vi "Chroma Driver GPIB-VISA-RW.vi"(0 "VISA resource name":refnum<visa-resource-name>="CHROMA", 5 "Chroma Power Select":T1, 9 "Write Buffer":string="SENS:DATA?", 11 "error in (no error)":errorcluster) -> (6 "Read Array":string[](array[string]), 15 "error out":errorcluster)   [LabVIEW 2012]
doc: "This example requires NI-488.2 and NI-VISA to be installed on the system. The example shows how to communicate with a GPIB instrument using VISA reads, writes, and formatting functions on the returned data. This example will work using an NI Instrument Simulator or other instrument that has similar behavior."
uses:
  Chroma Driver Select.ctl
  <vilib>/Instr/_visa.llb/VISA Open Access Mode.ctl
panel:
  out "Array":errorcluster[](array[cluster])
  out "Success":bool
  out "Read Buffer":string
  # "Voltage \nPower\nCurrent \nState\nPhase\nError?"
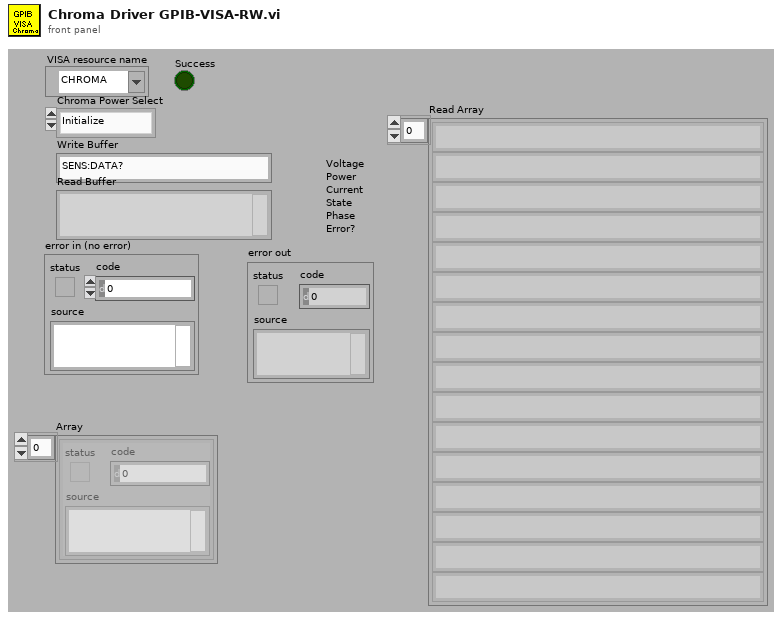
[diagram p1: front panel]
types:
  T1 = typedef "Chroma Driver Select.ctl" = enum16{"Initialize", "Output On 120", "Output On 240", "Output On 208", "Output Off", "Status", "Send Command", "Track Current"}
  T2 = typedef "VISA Open Access Mode.ctl" = u32
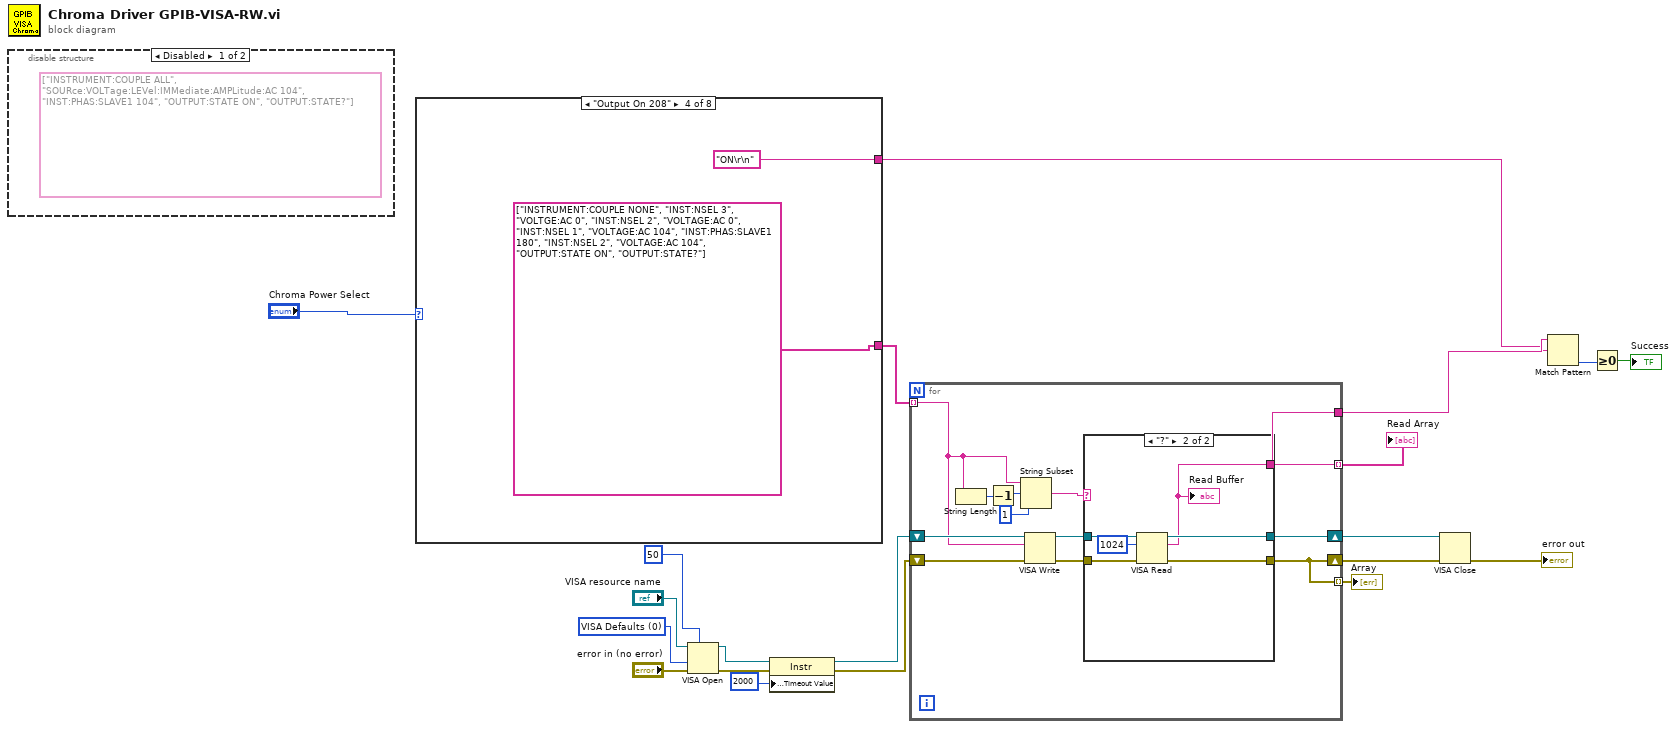
[diagram p0: block diagram]
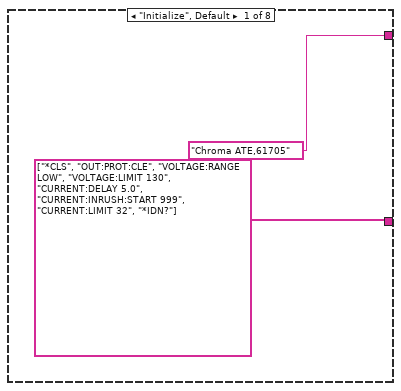
[diagram p4: hidden frame]
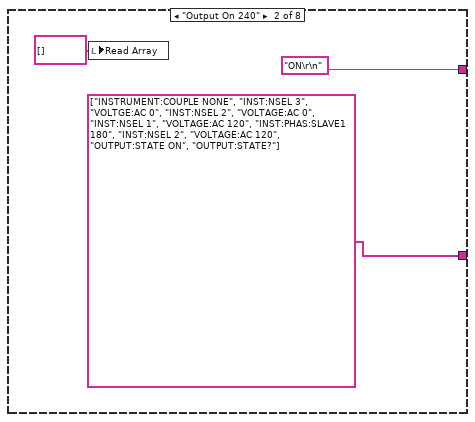
[diagram p5: hidden frame]
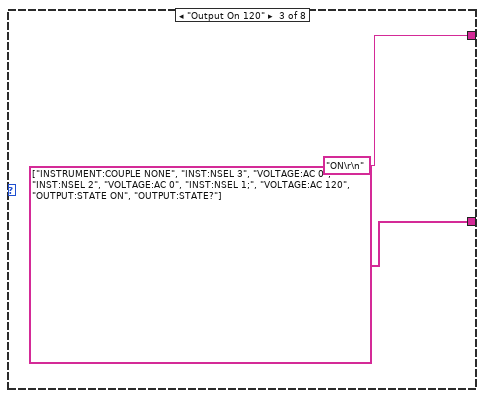
[diagram p6: hidden frame]
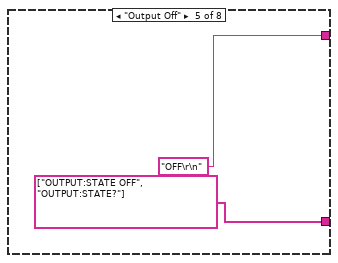
[diagram p7: hidden frame]
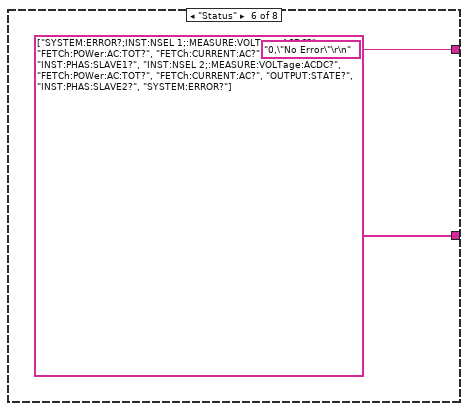
[diagram p8: hidden frame]
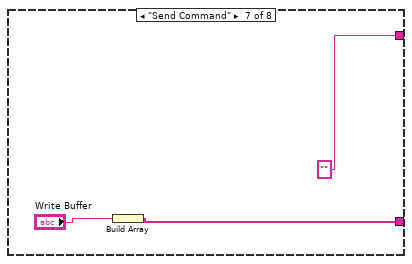
[diagram p9: hidden frame]
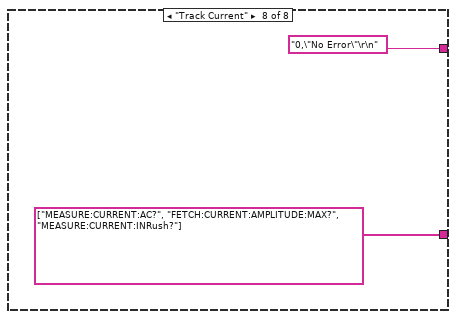
[diagram p10: hidden frame]
diagram:
  w14 = T2 0 items=["VISA Defaults"=0, "Exclusive Lock"=1, "Load Configured Settings"=4] ("Access Mode")
  n1 = disable-structure shown="Disabled" {
    frame Disabled {
      (unwired) string[] ["INSTRUMENT:COUPLE ALL", "SOURce:VOLTage:LEVel:IMMediate:AMPLitude:AC 104", "INST:PHAS:SLAVE1 104", "OUTPUT:STATE ON", "OUTPUT:STATE?"]
    }
    frame Enabled {
    }
  }
  n2 = case shown="\"Output On 208\"" "Chroma Power Select" {
    tunnel: [string[] ["*CLS", "OUT:PROT:CLE", "VOLTAGE:RANGE LOW", "VOLTAGE:LIMIT 130", "CURRENT:DELAY 5.0", "CURRENT:INRUSH:START 999", "CURRENT:LIMIT 32", "*IDN?"] string[] ["INSTRUMENT:COUPLE NONE", "INST:NSEL 3", "VOLTGE:AC 0", "INST:NSEL 2", "VOLTAGE:AC 0", "INST:NSEL 1", "VOLTAGE:AC 120", "INST:PHAS:SLAVE1 180", "INST:NSEL 2", "VOLTAGE:AC 120", "OUTPUT:STATE ON", "OUTPUT:STATE?"] string[] ["INSTRUMENT:COUPLE NONE", "INST:NSEL 3", "VOLTAGE:AC 0", "INST:NSEL 2", "VOLTAGE:AC 0", "INST:NSEL 1;", "VOLTAGE:AC 120", "OUTPUT:STATE ON", "OUTPUT:STATE?"] string[] ["INSTRUMENT:COUPLE NONE", "INST:NSEL 3", "VOLTGE:AC 0", "INST:NSEL 2", "VOLTAGE:AC 0", "INST:NSEL 1", "VOLTAGE:AC 104", "INST:PHAS:SLAVE1 180", "INST:NSEL 2", "VOLTAGE:AC 104", "OUTPUT:STATE ON", "OUTPUT:STATE?"] string[] ["OUTPUT:STATE OFF", "OUTPUT:STATE?"] string[] ["SYSTEM:ERROR?;INST:NSEL 1;:MEASURE:VOLTage:ACDC?", "FETCh:POWer:AC:TOT?", "FETCh:CURRENT:AC?", "OUTPUT:STATE?", "INST:PHAS:SLAVE1?", "INST:NSEL 2;:MEASURE:VOLTage:ACDC?", "FETCh:POWer:AC:TOT?", "FETCh:CURRENT:AC?", "OUTPUT:STATE?", "INST:PHAS:SLAVE2?", "SYSTEM:ERROR?"] w36 string[] ["MEASURE:CURRENT:AC?", "FETCH:CURRENT:AMPLITUDE:MAX?", "MEASURE:CURRENT:INRush?"]] -> w10
    tunnel: ["Chroma ATE,61705" ("string to write") "ON\r\n" ("read buffer") "ON\r\n" ("read buffer") "ON\r\n" ("read buffer") "OFF\r\n" ("read buffer") "0,\"No Error\"\r\n" ("string to write") "" ("Response") "0,\"No Error\"\r\n" ("string to write")] -> w1
    frame "Initialize", Default {
    }
    frame "Output On 240" {
      n3 = local write "Read Array"(string[] [] ("Read Array")) -> ()
    }
    frame "Output On 120" {
    }
    frame "Output On 208" {
    }
    frame "Output Off" {
    }
    frame "Status" {
    }
    frame "Send Command" {
      n4 = Build Array("Write Buffer") -> (w36:string[])
    }
    frame "Track Current" {
    }
  }
  n5 = VISA Open(timeout (0)=u32 50 ("VISA Open timeout (0)"), access mode=w14, error in (no error)="error in (no error)", VISA resource name="VISA resource name") -> (VISA resource name=w16:refnum<visa-resource-name>, error out=w15:errorcluster)  [unwired: 1 in]
  n6 = property class="Instr"(reference=w16, error in=w15, "General Settings:Timeout Value"=u32 2000) -> (reference out=w12:refnum<visa-resource-name>, error out=w13:errorcluster)
  n7 = for {
    tunnel: w10 -> [w44] mode=indexing
    shift-right: [w49] -> w20
    shift-left: w12 -> [w46]
    shift-right: [w39] -> w19
    shift-left: w13 -> [w47]
    tunnel: [w40] -> w7 mode=indexing
    tunnel: [w40] -> w2
    tunnel: [w39] -> w6 mode=indexing
    n8 = String Length(string=w44) -> (length=w42:i32)
    n9 = Decrement(x=w42) -> (x-1=w43:i32)
    n10 = String Subset(string=w44, offset (0)=w43, length (rest)=1 ("length (rest)")) -> (substring=w45:string)
    n11 = VISA Write(VISA resource name=w46, write buffer=w44, error in (no error)=w47) -> (VISA resource name out=w50:refnum<visa-resource-name>, error out=w48:errorcluster)  [unwired: 1 out]
    n12 = case shown="\"?\"" w45 {
      tunnel: w50 -> [w52 w58]
      tunnel: [w52 w57] -> w49
      tunnel: w48 -> [w51 w56]
      tunnel: [w51 w55] -> w39
      tunnel: [_ w53] -> w40
      frame "Not ?", Default {
      }
      frame "?" {
        n13 = VISA Read(VISA resource name=w58, byte count=u32 1024, error in (no error)=w56) -> (VISA resource name out=w57:refnum<visa-resource-name>, read buffer=w53:string, error out=w55:errorcluster)  [unwired: 1 out]
        "Read Buffer" <- w53
      }
    }
  }
  "Read Array" <- w7
  "Array" <- w6
  n14 = VISA Close(VISA resource name=w20, error in (no error)=w19) -> (error out=→"error out":errorcluster)
  n15 = Match Pattern(string=w2, regular expression=w1) -> (offset past match=w4:i32)  [unwired: 1 in, 3 out]
  n16 = Greater Or Equal To 0?(x=w4) -> (x >= 0?=→"Success":bool)
